vi "U8-Array to U64.vi"(10 "U8 Array":u8[](array[numeric])) -> (2 "U64 Array":u64[](array[numeric]))   [LabVIEW 2014, in "hse-misc.lvlib"]
doc: "Convert an array of Bytes (U8) to an array of U64."
uses:
  hse-misc.lvlib
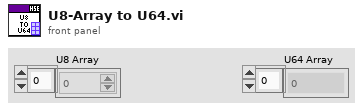
[diagram p1: front panel]
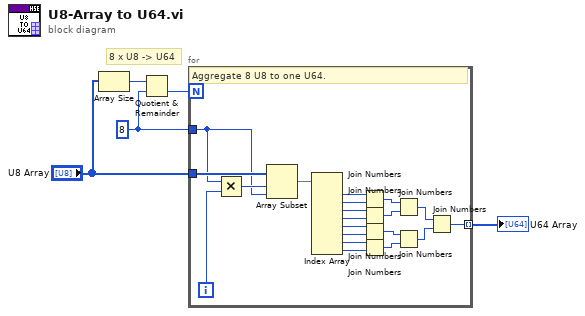
[diagram p0: block diagram]
diagram:
  w2 = 8 ("y")
  # "8 x U8 -> U64"
  n1 = Array Size(array="U8 Array") -> (size(s)=w4:i32)
  n2 = Quotient & Remainder(x=w4, y=w2) -> (floor(x/y)=w3:i32)  [unwired: 1 out]
  n3 = for {
    N: w3 -> [_]
    tunnel: "U8 Array" -> [w25]
    tunnel: w2 -> [w22]
    tunnel: [w6] -> w1 mode=indexing
    i -> [w24]
    # "Aggregate 8 U8 to one U64."
    n4 = Multiply(x=w22, y=w24) -> (x*y=w23:i32)
    n5 = Array Subset(array=w25, index=w23, length=w22) -> (w21:u8[])
    n6 = Index Array(array=w21) -> (element #1=w20:u8, element #2=w19:u8, element #3=w18:u8, element #4=w17:u8, element #5=w16:u8, element #6=w15:u8, element #7=w14:u8, element #8=w13:u8)  [unwired: 8 in]
    n7 = Join Numbers(hi=w20, lo=w19) -> ((hi.lo)=w12:u16)
    n8 = Join Numbers(hi=w18, lo=w17) -> ((hi.lo)=w11:u16)
    n9 = Join Numbers(hi=w16, lo=w15) -> ((hi.lo)=w10:u16)
    n10 = Join Numbers(hi=w14, lo=w13) -> ((hi.lo)=w9:u16)
    n11 = Join Numbers(hi=w12, lo=w11) -> ((hi.lo)=w8:u32)
    n12 = Join Numbers(hi=w10, lo=w9) -> ((hi.lo)=w7:u32)
    n13 = Join Numbers(hi=w8, lo=w7) -> ((hi.lo)=w6:u64)
  }
  "U64 Array" <- w1
